vi "FTW-CodeGen-Prototype.vi"(5 "REPLACE_UpstreamTime":dbl=-1.0 format="%.4psec") -> (4 "REPLACE_HiResTimer":dbl format="%.4psec", 6 "REPLACE_HiResElapsedTime":dbl format="%.4psec")   [LabVIEW 2014, in "FTW-Dataflow-Synchronizer.xnode"]
uses:
  FTW-Dataflow-Synchronizer.xnode
panel:
  # "Inputs"
  # "Outputs"
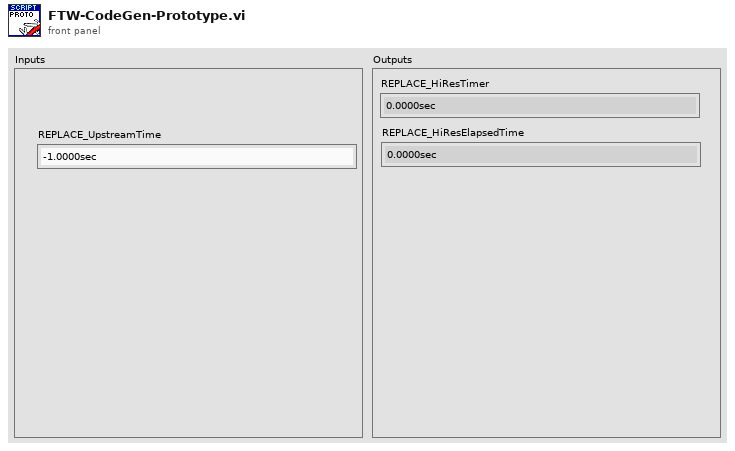
[diagram p1: front panel]
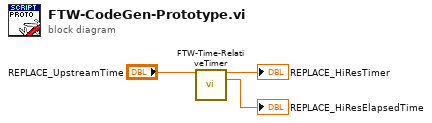
[diagram p0: block diagram]
diagram:
  n1 = call "FTW-Time-RelativeTimer.vi"("Previous Timer Value"="REPLACE_UpstreamTime") -> ("Current Timer Value"=→"REPLACE_HiResTimer":dbl, "Elapsed Time"=→"REPLACE_HiResElapsedTime":dbl)  [unwired: 12 in, 1 out]
